vi "New2-Track.vi"(0 "vid bandpass":T1, 1 "mask":bool[][](array[boolean]), 2 "# of logical processors":i32, 5 "correct":dbl[](array[numeric]), 7 "incorrect":dbl[](array[numeric]), 9 "exit rad":dbl, 12 "X Resolution":i32, 13 "Y Resolution":i32, 14 "Image Pixels (U8)":u8[][](array[numeric])) -> (4 "%inexit":dbl[](array[numeric]), 6 "centroid":dbl[](array[numeric]), 10 "Numeric":i32, 15 "vid":u8[][](array[numeric]))   [LabVIEW 2019]
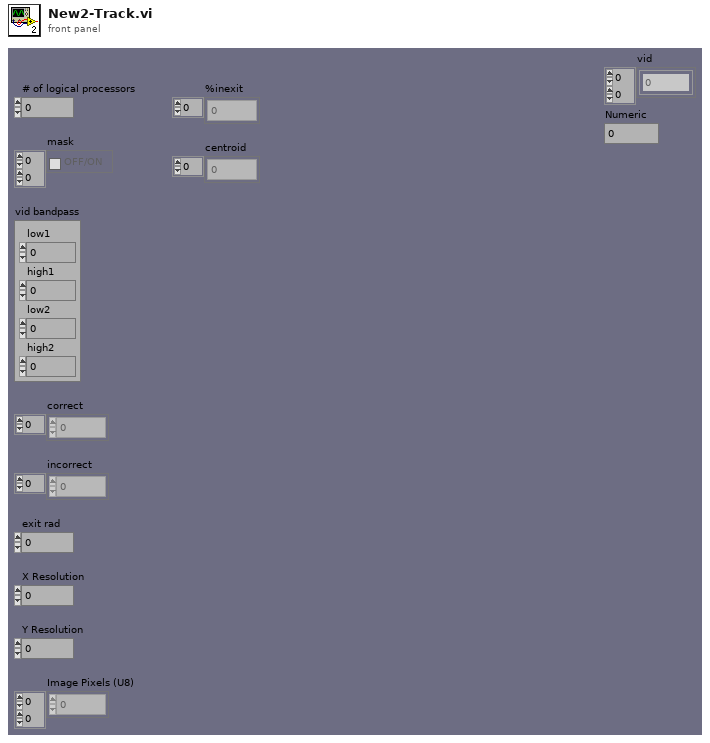
[diagram p1: front panel]
types:
  T1 = cluster{"low1":i32, "high1":i32, "low2":i32, "high2":i32}
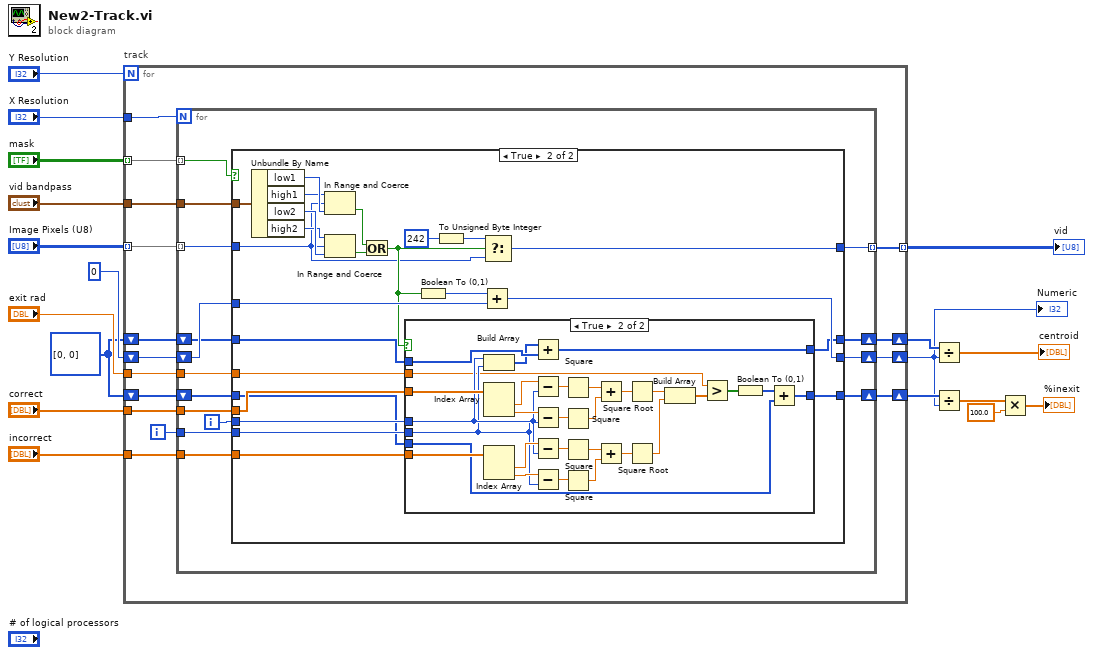
[diagram p0: block diagram]
diagram:
  w1 = i32[] [0, 0]
  n1 = for "track" {
    N: "Y Resolution" -> [_]
    tunnel: "exit rad" -> [w29]
    tunnel: "correct" -> [w28]
    tunnel: "X Resolution" -> [w33]
    tunnel: "mask" -> [w32] mode=indexing
    tunnel: "Image Pixels (U8)" -> [w31] mode=indexing
    tunnel: "vid bandpass" -> [w30]
    tunnel: "incorrect" -> [w26]
    shift-right: [w25] -> w3
    shift-left: 0 -> [w24]
    shift-right: [w23] -> w7
    shift-left: w1 -> [w22]
    tunnel: [w21] -> w6 mode=indexing
    shift-right: [w20] -> w4
    shift-left: w1 -> [w19]
    i -> [w27]
    n2 = for {
      N: w33 -> [_]
      tunnel: w32 -> [w42] mode=indexing
      tunnel: w31 -> [w48] mode=indexing
      tunnel: w30 -> [w47]
      tunnel: w29 -> [w46]
      tunnel: w28 -> [w45]
      tunnel: w27 -> [w43]
      tunnel: w26 -> [w41]
      shift-right: [w40] -> w25
      shift-left: w24 -> [w39]
      shift-right: [w38] -> w23
      shift-left: w22 -> [w37]
      tunnel: [w36] -> w21 mode=indexing
      shift-right: [w35] -> w20
      shift-left: w19 -> [w34]
      i -> [w44]
      n3 = case shown="True" w42 {
        tunnel: w48 -> [w50 w61]
        tunnel: w47 -> [_ w69]
        tunnel: w46 -> [_ w68]
        tunnel: w45 -> [_ w70]
        tunnel: w44 -> [_ w57]
        tunnel: w43 -> [_ w56]
        tunnel: w41 -> [_ w67]
        tunnel: [w52 w65] -> w40
        tunnel: w39 -> [w52 w64]
        tunnel: [w51 w58] -> w38
        tunnel: w37 -> [w51 w59]
        tunnel: [w50 w60] -> w36
        tunnel: [w49 w55] -> w35
        tunnel: w34 -> [w49 w54]
        frame False {
        }
        frame True {
          n4 = Unbundle By Name(w69) -> ("low1"=w76:i32, "high1"=w75:i32, "low2"=w74:i32, "high2"=w73:i32)
          n5 = In Range and Coerce(upper limit=w75, x=w61, lower limit=w76) -> (In Range?=w72:bool)  [unwired: 1 out]
          n6 = In Range and Coerce(upper limit=w73, x=w61, lower limit=w74) -> (In Range?=w71:bool)  [unwired: 1 out]
          n7 = Or(x=w72, y=w71) -> (x .or. y?=w63:bool)
          n8 = case shown="True" w63 {
            tunnel: w70 -> [_ w107]
            tunnel: w68 -> [_ w83]
            tunnel: w67 -> [_ w106]
            tunnel: w59 -> [w78 w105]
            tunnel: [w78 w104] -> w58
            tunnel: w57 -> [_ w88]
            tunnel: w56 -> [_ w87]
            tunnel: [w77 w80] -> w55
            tunnel: w54 -> [w77 w79]
            frame False {
            }
            frame True {
              n9 = Build Array(w88, w87) -> (w89:i32[])
              n10 = Index Array(array=w107) -> (element #1=w102:dbl, element #2=w103:dbl)  [unwired: 2 in]
              n11 = Index Array(array=w106) -> (element #1=w95:dbl, element #2=w96:dbl)  [unwired: 2 in]
              n12 = Add(x=w89, y=w105) -> (x+y=w104:i32[])
              n13 = Subtract(x=w102, y=w88) -> (x-y=w97:dbl)
              n14 = Subtract(x=w103, y=w87) -> (x-y=w98:dbl)
              n15 = Subtract(x=w95, y=w88) -> (x-y=w90:dbl)
              n16 = Subtract(x=w96, y=w87) -> (x-y=w91:dbl)
              n17 = Square(x=w97) -> (x^2=w99:dbl)
              n18 = Square(x=w98) -> (x^2=w100:dbl)
              n19 = Square(x=w90) -> (x^2=w92:dbl)
              n20 = Square(x=w91) -> (x^2=w93:dbl)
              n21 = Add(x=w99, y=w100) -> (x+y=w101:dbl)
              n22 = Add(x=w92, y=w93) -> (x+y=w94:dbl)
              n23 = Square Root(x=w101) -> (sqrt(x)=w86:dbl)
              n24 = Square Root(x=w94) -> (sqrt(x)=w85:dbl)
              n25 = Build Array(w86, w85) -> (w84:dbl[])
              n26 = Greater?(x=w83, y=w84) -> (0:w82:bool[])
              n27 = Boolean To (0,1)(Boolean=w82) -> (0, 1=w81:i16[])
              n28 = Add(x=w81, y=w79) -> (x+y=w80:i32[])
            }
          }
          n29 = Boolean To (0,1)(Boolean=w63) -> (0, 1=w66:i16)
          n30 = To Unsigned Byte Integer(number=242) -> (unsigned 8bit integer=w53:u8)
          n31 = Add(x=w66, y=w64) -> (x+y=w65:i32)
          n32 = Select(t=w53, s=w63, f=w61) -> (s? t:f=w60:u8)
        }
      }
    }
  }
  "vid" <- w6
  "Numeric" <- w3
  n33 = Divide(x=w7, y=w3) -> (x/y=→"centroid":dbl[])
  n34 = Divide(x=w4, y=w3) -> (x/y=w2:dbl[])
  n35 = Multiply(x=w2, y=100.0) -> (x*y=→"%inexit":dbl[])
